vi "wait for SOMD ready.vi"(0 "USB":i32, 1 "WaitTime":i32=100 caption="Time to Wait [ms]" min=0 max=10000 step=50, 2 "Max Loops":i32 min=-1 max=1000 step=1, 5 "SLOT":i32=100, 7 "InpRefToOutput":refnum<vi>, 9 "Stopp":bool, 11 "error in (no error)":errorcluster caption="Error IN", 12 "Exit On HWErrors":bool, 13 "State Check Mask":u16 format="%04x") -> (4 "Final State":u16 format="%04x", 6 "Loops On Exit":i32 min=-1 max=999 step=1, 8 "Exiting with HWError":bool caption="with HWError", 10 "HW Ready to Run":bool caption="Ready to Run", 15 "error out":errorcluster caption="Error OUT")   [LabVIEW 2020]
panel:
  out "OutputRef":refnum<vi>
  out "Substitute Output":string caption="Substit. Output (if InpRef is invalid)"
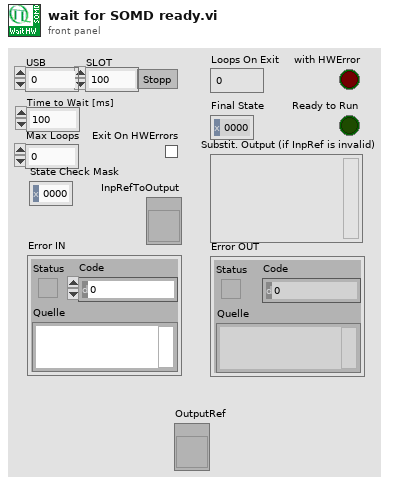
[diagram p1: front panel]
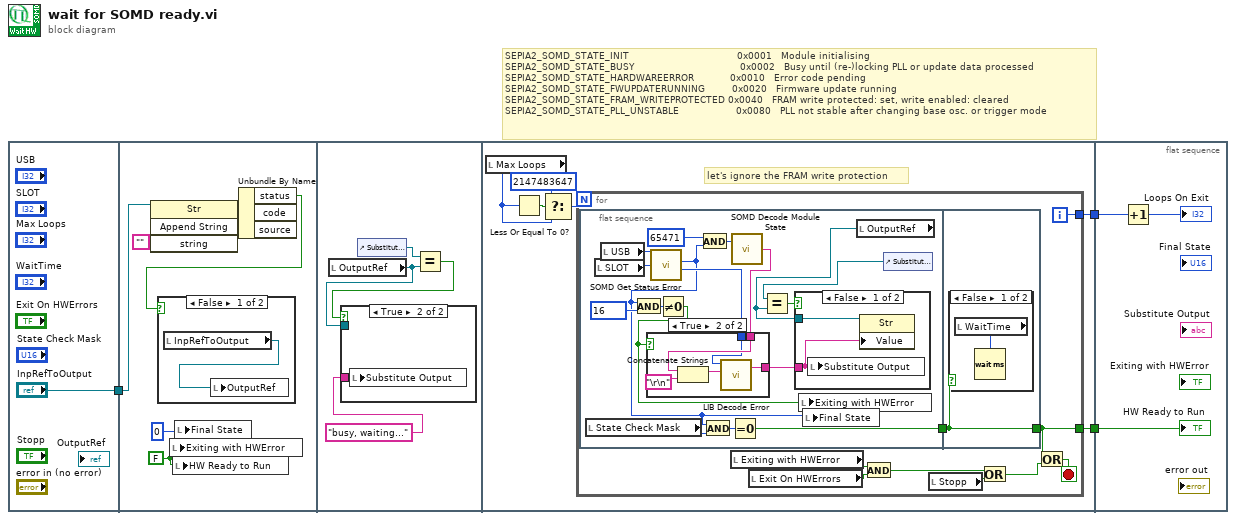
[diagram p0: block diagram]
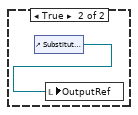
[diagram p2: hidden frame]
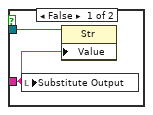
[diagram p3: hidden frame]
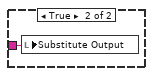
[diagram p4: hidden frame]
diagram:
  # "SEPIA2_SOMD_STATE_INIT                                    0x0001   Module initialising\nSEPIA2_SOMD_STATE_BUSY                                   0x0002   Busy until (re-)locking PLL or update data processed\nSEPIA2_SOMD_STATE_HARDWAREERROR            0x0010   Error code pending\nSEPIA2_SOMD_STATE_FWUPDATERUNNING         0x0020   Firmware update running\nSEPIA2_SOMD_STATE_FRAM_WRITEPROTECTED 0x0040   FRAM write protected: set, write enabled: cleared\nSEPIA2_SOMD_STATE_PLL_UNSTABLE                   0x0080   PLL not stable after changing base osc. or trigger mode"
  n1 = flat-sequence {
    tunnel: ["InpRefToOutput"] -> w1
    tunnel: w1 -> [w10]
    tunnel: [w22] -> w3
    tunnel: [w21] -> w2
    tunnel: w3 -> [w64]
    tunnel: w2 -> [w63]
    frame #0 {
    }
    frame #1 {
      w6 = FALSE
      n2 = invoke class="Str" method="Append String"(reference=w10, "string"="") -> (error out=w8:errorcluster)  [unwired: 2 in, 3 out]
      n3 = local write "Exiting with HWError"(w6) -> ()
      n4 = local write "HW Ready to Run"(w6) -> ()
      n5 = local write "Final State"(u16 0) -> ()
      n6 = Unbundle By Name(w8) -> ("status"=w7:bool)  [unwired: 2 out]
      n7 = case shown="False" w7 {
        frame False {
          n8 = local read "InpRefToOutput"() -> (w11:refnum<vi>)
          n9 = local write "OutputRef"(w11) -> ()
        }
        frame True {
          n10 = control-ref of="Substitute Output"() -> (w12:refnum<vi>)
          n11 = local write "OutputRef"(w12) -> ()
        }
      }
    }
    frame #2 {
      n12 = local read "OutputRef"() -> (w15:refnum<vi>)
      n13 = control-ref of="Substitute Output"() -> (w14:refnum<vi>)
      n14 = Equal?(x=w14, y=w15) -> (x = y?=w13:bool)
      n15 = case shown="True" w13 {
        tunnel: "busy, waiting..." -> [w18 w19]
        tunnel: w15 -> [w17 _]
        frame False {
          n16 = local write "Substitute Output"(w18) -> ()
          n17 = property class="Str"(reference=w17, "Value"=w18) -> ()  [unwired: 1 in, 2 out]
        }
        frame True {
          n18 = local write "Substitute Output"(w19) -> ()
        }
      }
    }
    frame #3 {
      # "let's ignore the FRAM write protection"
      n19 = local read "Max Loops"() -> (w20:i32)
      n20 = Less Or Equal To 0?(x=w20) -> (x <= 0?=w25:bool)
      n21 = Select(t=2147483647, s=w25, f=w20) -> (s? t:f=w24:i32)
      n22 = for {
        N: w24 -> [_]
        tunnel: [w34] -> w22
        tunnel: [w27] -> w21
        i -> [w34]
        stop <- w30 stop-if-true
        n23 = flat-sequence {
          tunnel: [w45] -> w26
          tunnel: [w61] -> w27
          tunnel: w26 -> [w61]
          frame #0 {
            n24 = local read "State Check Mask"() -> (w44:u16)
            n25 = local read "SLOT"() -> (w51:i32)
            n26 = local read "USB"() -> (w50:i32)
            n27 = call "SOMD Get Status Error.vi"("DevIdx"=w50, "SlotId"=w51) -> ("Module State"=w35:u16, "Error Code"=w43:i16)  [unwired: 1 in, 2 out]
            n28 = And(x=w35, y=u16 16) -> (x .and. y?=w48:u16)
            n29 = Not Equal To 0?(x=w48) -> (x != 0?=w40:bool)
            n30 = And(x=u16 65471, y=w35) -> (x .and. y?=w42:u16)
            n31 = And(x=w35, y=w44) -> (x .and. y?=w46:u16)
            n32 = Equal To 0?(x=w46) -> (x = 0?=w45:bool)
            n33 = call "SOMD Decode Module State.vi"("Module State Code"=w42) -> ("Module State"=w47:string)  [unwired: 1 in, 2 out]
            n34 = case shown="True" w40 {
              tunnel: [w55 w60] -> w36
              tunnel: w47 -> [w55 w59]
              tunnel: w43 -> [_ w56]
              frame False {
              }
              frame True {
                n35 = Concatenate Strings(w59, "\r\n") -> (w58:string)
                n36 = call "LIB Decode Error.vi"("error source (\" \")"=w58, "error code"=w56) -> ("error txt"=w60:string)  [unwired: 2 in, 1 out]
              }
            }
            n37 = local write "Exiting with HWError"(w40) -> ()
            n38 = local write "Final State"(w35) -> ()
            n39 = local read "OutputRef"() -> (w38:refnum<vi>)
            n40 = control-ref of="Substitute Output"() -> (w37:refnum<vi>)
            n41 = Equal?(x=w37, y=w38) -> (x = y?=w39:bool)
            n42 = case shown="False" w39 {
              tunnel: w38 -> [w53 _]
              tunnel: w36 -> [w52 w54]
              frame False {
                n43 = local write "Substitute Output"(w52) -> ()
                n44 = property class="Str"(reference=w53, "Value"=w52) -> ()  [unwired: 1 in, 2 out]
              }
              frame True {
                n45 = local write "Substitute Output"(w54) -> ()
              }
            }
          }
          frame #1 {
            n46 = case shown="False" w61 {
              frame False {
                n47 = local read "WaitTime"() -> (w62:i32)
                n48 = Wait (ms)(milliseconds to wait=w62) -> ()  [unwired: 1 out]
              }
              frame True {
              }
            }
          }
        }
        n49 = local read "Exiting with HWError"() -> (w31:bool)
        n50 = local read "Exit On HWErrors"() -> (w32:bool)
        n51 = And(x=w31, y=w32) -> (x .and. y?=w28:bool)
        n52 = local read "Stopp"() -> (w33:bool)
        n53 = Or(x=w28, y=w33) -> (x .or. y?=w29:bool)
        n54 = Or(x=w27, y=w29) -> (x .or. y?=w30:bool)
      }
    }
    frame #4 {
      n55 = Increment(x=w64) -> (x+1=→"Loops On Exit":i32)
      "HW Ready to Run" <- w63
    }
  }
